vi "Resolve API URL.vi"(11 "API URL":string) -> (3 "result string":string)   [LabVIEW 2024]
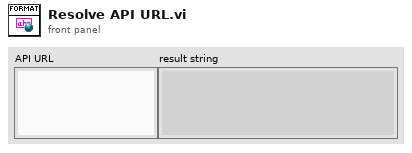
[diagram p1: front panel]
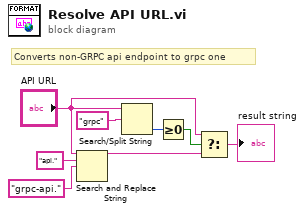
[diagram p0: block diagram]
diagram:
  # "Converts non-GRPC api endpoint to grpc one"
  n1 = Search and Replace String(input string="API URL", search string="api.", replace string="grpc-api." ("replace string (\"\")")) -> (result string=w3:string)  [unwired: 5 in, 3 out]
  n2 = Search/Split String(string="API URL", search string/char (-)="grpc") -> (offset of match=w5:i32)  [unwired: 1 in, 2 out]
  n3 = Greater Or Equal To 0?(x=w5) -> (x >= 0?=w4:bool)
  n4 = Select(t="API URL", s=w4, f=w3) -> (s? t:f=→"result string":string)
